vi "Format_and_Increment_Indices.vi"(4 "error in":errorcluster, 5 "Indices":i32[](array[numeric]), 6 "DimSizes":i32[](array[numeric]), 7 "initial string":string) -> (0 "error out":errorcluster, 1 "New Indices":i32[](array[numeric]), 3 "string w/ indices":string)   [LabVIEW 2011, in "Third Party VIs.lvlib" / "pcardinale.lvlib"]
doc: "Formats indices into string.\nAdvances indices to next element."
uses:
  pcardinale.lvlib
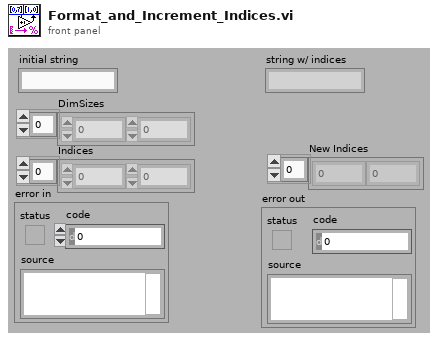
[diagram p1: front panel]
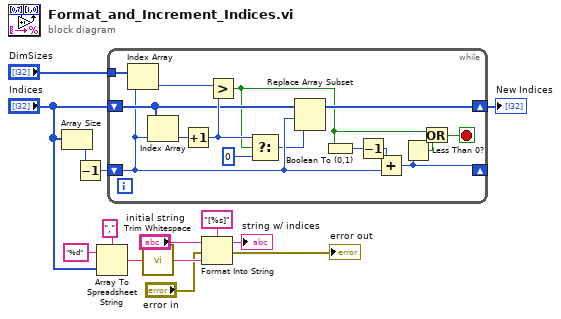
[diagram p0: block diagram]
diagram:
  n1 = Array Size(array="Indices") -> (size(s)=w8:i32)
  n2 = Decrement(x=w8) -> (x-1=w6:i32)
  n3 = Array To Spreadsheet String(delimiter (Tab)=",", array="Indices", 3:"%d" ("format string")) -> (spreadsheet string=w12:string)
  n4 = while {
    shift-right: [w21] -> _
    shift-left: w6 -> [w17]
    tunnel: "DimSizes" -> [w28]
    shift-right: [w24] -> w5
    shift-left: "Indices" -> [w25]
    stop <- w19 stop-if-true
    n5 = Index Array(array=w28, index=w17) -> (element=w18:i32)
    n6 = Index Array(array=w25, index=w17) -> (element=w29:i32)
    n7 = Increment(x=w29) -> (x+1=w27:i32)
    n8 = Greater?(x=w18, y=w27) -> (0:w15:bool)
    n9 = Select(t=w27, s=w15, f=0) -> (s? t:f=w16:i32)
    n10 = Replace Array Subset(array=w25, new element=w16, index=w17) -> (w24:i32[])
    n11 = Boolean To (0,1)(Boolean=w15) -> (0, 1=w23:i16)
    n12 = Decrement(x=w23) -> (x-1=w22:i16)
    n13 = Add(x=w22, y=w17) -> (x+y=w21:i32)
    n14 = Less Than 0?(x=w21) -> (x < 0?=w20:bool)
    n15 = Or(x=w15, y=w20) -> (x .or. y?=w19:bool)
  }
  "New Indices" <- w5
  n16 = call <vilib>:"Trim Whitespace.vi"("string"=w12) -> ("trimmed string"=w4:string)  [unwired: 1 in]
  n17 = Format Into String(format string="[%s]", initial string="initial string", error in="error in", w4) -> (resulting string=→"string w/ indices":string, error out=→"error out":errorcluster)
